vi "Set Segmenting Specification.vi"   [LabVIEW 2020, in "NI_VS Data Logging API.lvlib"]
doc: "Specifies how to segment the log files created during the data logging session. You can segment log files according to time or size limits, or when a start trigger occurs. When the segmenting condition is met, this VI saves and closes the current log file and continues logging data in a new file.\n\nSelect the Default instance of this VI if you do not want to segment log files based on time or size, but do want the option to segment on a start trigger.\n\nYou must manually select the polymorphic instance to use."
uses:
  <vilib>/NI VeriStand/Execution/DataLogging/NI_VS Data Logging API.lvlib
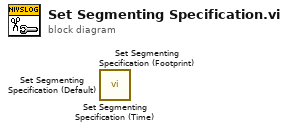
[diagram p0: block diagram]
diagram:
  n1 = call <vilib>:"Set Segmenting Specification (Time).vi"() -> ()  [unwired: 10 in, 2 out]
  n2 = call <vilib>:"Set Segmenting Specification (Footprint).vi"() -> ()  [unwired: 10 in, 2 out]
  n3 = call <vilib>:"Set Segmenting Specification (Default).vi"() -> ()  [unwired: 10 in, 2 out]
